vi "_Copy 1.vi"(0 "XRef":T5, 1 "State In":T1) -> (14 "Reply":T3, 15 "Fatal Error Out":T2, 16 "State Out":T1)   [LabVIEW 2014, in "JKISM++ Explorer to Example.xnode"]
uses:
  JKISM++ Explorer to Example.xnode
  <vilib>/XNodeSupport/XNodeXNodeRef.ctl
  _State 1.ctl
  <vilib>/XNodeSupport/XNodeStringArray.ctl
  <vilib>/XNodeSupport/XNodeString.ctl
  <vilib>/XNodeSupport/XNodeErrorCluster.ctl
  <vilib>/XNodeSupport/NI_XNodeSupport.lvlib
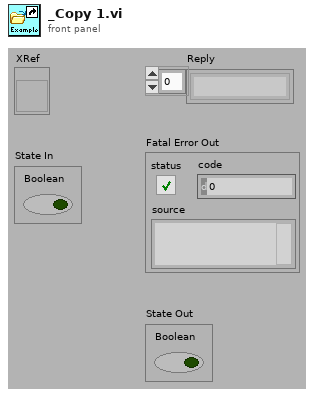
[diagram p1: front panel]
types:
  T1 = typedef "JKISM++ Explorer to Example.xnode/_State 1.ctl" = cluster{"Boolean":bool}
  T2 = typedef "NI_XNodeSupport.lvlib/XNodeErrorCluster.ctl" = errorcluster
  T3 = typedef "NI_XNodeSupport.lvlib/XNodeStringArray.ctl" = T4[]
  T4 = typedef "NI_XNodeSupport.lvlib/XNodeString.ctl" = string
  T5 = typedef "NI_XNodeSupport.lvlib/XNodeXNodeRef.ctl" = refnum<vi>
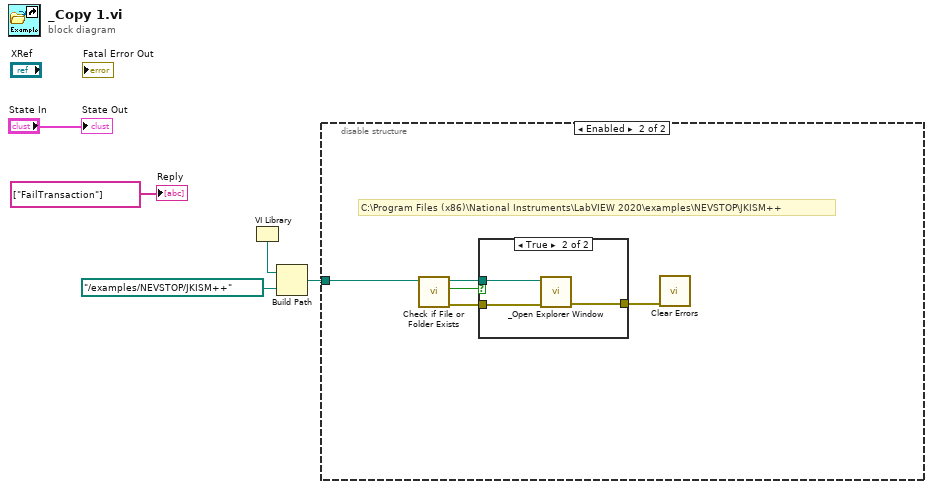
[diagram p0: block diagram]
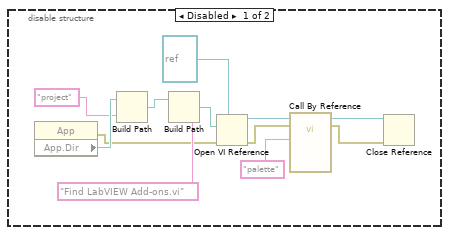
[diagram p2: hidden frame]
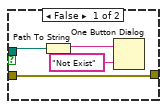
[diagram p3: hidden frame]
diagram:
  n1 = VI Library() -> (path=w1:path)
  n2 = Build Path(base path=w1, name or relative path=path "../examples/NEVSTOP/JKISM++" ("Relative path (.)")) -> (appended path=w2:path)
  n3 = disable-structure shown="Enabled" {
    disable-tunnel: w2 -> [_ w21]
    frame Disabled {
      n4 = property class="App"() -> (error out=w12:errorcluster, "App.Dir"=w17:path)  [unwired: 2 in, 1 out]
      n5 = Build Path(base path=w17, name or relative path="project") -> (appended path=w15:path)
      n6 = Build Path(base path=w15, name or relative path="Find LabVIEW Add-ons.vi") -> (appended path=w13:path)
      n7 = Open VI Reference(type specifier VI Refnum (for type only)=refnum<vi> refnum ("reference"), vi path=w13, error in (no error)=w12) -> (vi reference=w10:refnum<vi>, error out=w7:errorcluster)  [unwired: 3 in]
      n8 = call-by-ref "?"(reference=w10, error in=w7, "Source"="palette") -> (reference out=w6:refnum<vi>, error out=w8:errorcluster)  [unwired: 11 in]
      n9 = Close Reference(reference=w6, error in (no error)=w8) -> ()  [unwired: 1 out]
    }
    frame Enabled {
      # "C:\\Program Files (x86)\\National Instruments\\LabVIEW 2020\\examples\\NEVSTOP\\JKISM++"
      n10 = call <vilib>:"Check if File or Folder Exists.vi"("path"=w21) -> ("error out"=w19:errorcluster, "file or folder exists?"=w18:bool, "dup path"=w20:path)  [unwired: 8 in]
      n11 = case shown="True" w18 {
        tunnel: [w26 w29] -> w22
        tunnel: w20 -> [w25 w28]
        tunnel: w19 -> [w26 w27]
        frame False {
          n12 = Path To String(path=w25) -> (string=w24:string)
          n13 = One Button Dialog(message=w24, button name ("OK")="Not Exist") -> ()  [unwired: 1 out]
        }
        frame True {
          n14 = call "_Open Explorer Window.vi"("error in (no error)"=w27, "Directory or File"=w28) -> ("error out"=w29:errorcluster)  [unwired: 9 in]
        }
      }
      n15 = call <vilib>:"Clear Errors.vi"("error in (no error)"=w22) -> ()  [unwired: 6 in, 1 out]
    }
  }
  "Reply" <- T3 ["FailTransaction"] ("Reply")
  "State Out" <- "State In"
